vi "GetPressure.vi"(8 "error in (no error)":errorcluster, 11 "MKS999 in":refnum<class "MKS999.lvclass">) -> (0 "error out":errorcluster, 2 "Pressure (mbar)":dbl, 3 "MKS999 out":refnum<class "MKS999.lvclass">)   [LabVIEW 2016, in "MKS999.lvlib" / "MKS999.lvclass"]
uses:
  MKS999.lvclass
  MKS999.lvclass/MKS999.ctl
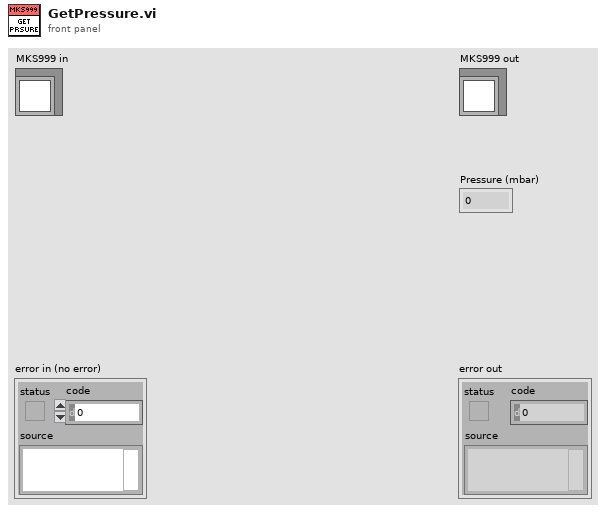
[diagram p1: front panel]
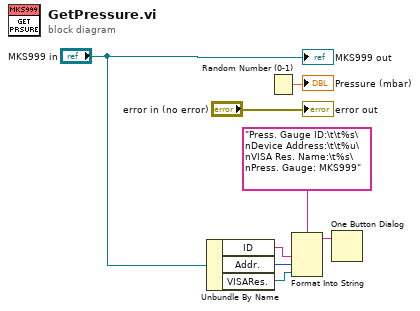
[diagram p0: block diagram]
diagram:
  n1 = Unbundle By Name("MKS999 in") -> ("ID"=w5:string, "Addr."=w6:u8, "VISARes."=w4:refnum<visa-resource-name>)
  n2 = Random Number (0-1)() -> (number: 0 to 1=→"Pressure (mbar)":dbl)
  n3 = Format Into String(format string="Press. Gauge ID:\t\t%s\nDevice Address:\t\t%u\nVISA Res. Name:\t%s\nPress. Gauge: MKS999", w5, w6, w4) -> (resulting string=w3:string)  [unwired: 2 in, 1 out]
  n4 = One Button Dialog(message=w3) -> ()  [unwired: 1 in, 1 out]
  "error out" <- "error in (no error)"
  "MKS999 out" <- "MKS999 in"
